vi "Process.vi"(8 "error in":errorcluster, 11 "Plugin in":refnum<class "Power Spectrum Density.lvclass">) -> (0 "error out":errorcluster, 3 "Plugin out":refnum<class "Power Spectrum Density.lvclass">)   [LabVIEW 2023, in "Power Spectrum Density.lvlib" / "Power Spectrum Density.lvclass"]
uses:
  Power Spectrum Density.lvclass
  Power Spectrum Density.lvclass/Power Spectrum Density.ctl
  Buffer Manager Function.ctl
  <vilib>/FlexLogger/SDK/PluginSDK.lvlibp/PEFClasses/SDK/Plugin/Plugin.lvclass
  C:/Program Files/National Instruments/LabVIEW 2023/vi.lib/FlexLogger/SDK/PluginSDK.lvlibp/PEFClasses/SDK/Plugin/Plugin.lvclass
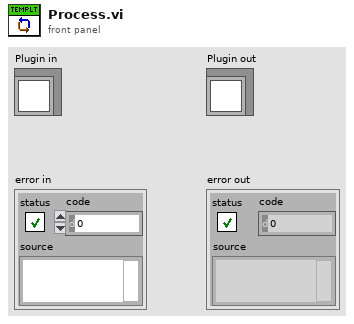
[diagram p1: front panel]
types:
  T1 = typedef "Power Spectrum Density.lvlib/Power Spectrum Density.lvclass/Buffer Manager Function.ctl" = enum16{"Get Data", "Buffer Data", "Reset Data"}
  T2 = typedef "Power Spectrum Density.lvlib/Power Spectrum Density.lvclass/Power Spectrum Density Data.ctl" = cluster{"First Time":bool, "Show PSD Window":bool, "Show PSD Window Clicked":bool, "Export mode":T3, "Window":T4, "dB":bool, "Averaging parameters":cluster{"averaging mode":enum16{"No averaging", "Vector averaging", "RMS averaging", "Peak hold"}, "weighting mode":enum16{"Linear", "Exponential"}, "number of averages":u32}, "Window parameter":dbl, "Number of Samples":i32, "PSD VI Ref":refnum<vi>}
  T3 = typedef "NI_MAPro.lvlib/Power Spectrum and PSD Export Mode.ctl" = u16
  T4 = typedef "NI_AALPro.lvlib/windowTd.ctl" = u32
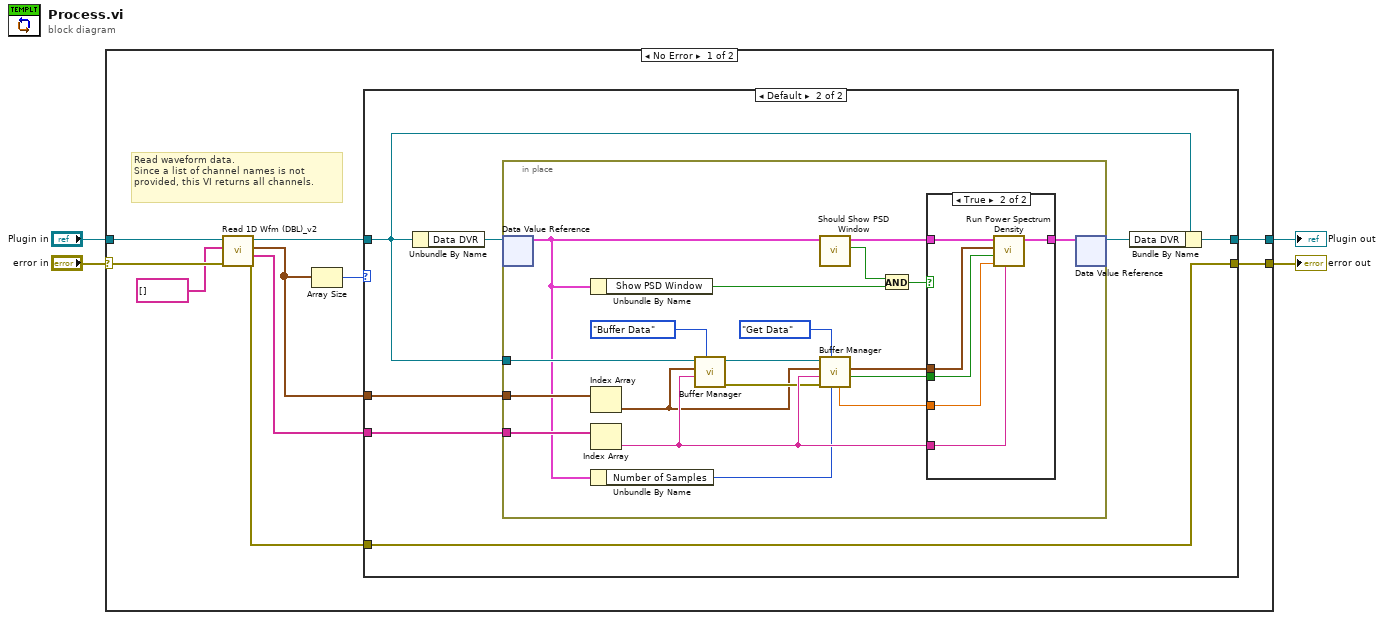
[diagram p0: block diagram]
diagram:
  n1 = case shown="No Error" "error in" {
    selector: "error in" -> [w13 w50]
    tunnel: [w11 w51] -> w3
    tunnel: "Plugin in" -> [w14 w51]
    tunnel: [w12 w50] -> w2
    frame No Error {
      # "Read waveform data.\nSince a list of channel names is not provided, this VI returns all channels."
      n2 = call <vilib>:"Read 1D Wfm (DBL)_v2.vi"("error in (no error)"=w13, "Unique Identifers (empty = all)"=string[] [] ("Unique Channel Identifers (empty = all)"), "Plugin in"=w14) -> ("error out"=w7:errorcluster, "Stream Names"=w5:string[], "Data"=w10:waveform(dbl)[], "Plugin out"=w8:refnum<class "Power Spectrum Density.lvclass">)  [unwired: 5 in]
      n3 = Array Size(array=w10) -> (size(s)=w9:i32)
      n4 = case shown="Default" w9 {
        tunnel: w10 -> [_ w23]
        tunnel: [w15 w22] -> w12
        tunnel: [w16 w18] -> w11
        tunnel: w8 -> [w16 w17]
        tunnel: w7 -> [w15 w22]
        tunnel: w5 -> [_ w21]
        frame 0 {
          # "No channels sending data to the plugin"
        }
        frame Default {
          n5 = Unbundle By Name(w17) -> ("Data DVR"=w20:refnum<data-value>)
          n6 = in-place {
            in-place-border: w23 -> [w40]
            in-place-border: w21 -> [w37]
            in-place-border: w17 -> [w39]
            n7 = in-place-dvr #1(w20) -> (w32:T2)  [unwired: 1 out]
            n8 = Unbundle By Name(w32) -> ("Show PSD Window"=w27:bool)
            n9 = Index Array(array=w40) -> (element=w29:waveform(dbl))  [unwired: 1 in]
            n10 = Index Array(array=w37) -> (element=w35:string)  [unwired: 1 in]
            n11 = Unbundle By Name(w32) -> ("Number of Samples"=w33:i32)
            n12 = call-dynamic "Buffer Manager.vi"("Function"=Buffer_Manager_Function."Buffer Data", "Unique Channel Identifier"=w35, "Waveform in"=w29, "Plugin in"=w39) -> ("error out"=w34:errorcluster, "Plugin out"=w36:refnum<class "Power Spectrum Density.lvclass">)  [unwired: 3 in, 3 out]
            n13 = call "Should Show PSD Window.vi"("Data in"=w32) -> ("Show window"=w26:bool, "Data out"=w42:T2)  [unwired: 9 in]
            n14 = call-dynamic "Buffer Manager.vi"("Number of Samples"=w33, "Function"=Buffer_Manager_Function."Get Data", "error in"=w34, "Unique Channel Identifier"=w35, "Waveform in"=w29, "Plugin in"=w36) -> ("Data Valid"=w25:bool, "Waveform out"=w28:waveform(dbl), "Percentage"=w24:dbl)  [unwired: 1 in, 2 out]
            n15 = And(x=w26, y=w27) -> (x .and. y?=w30:bool)
            n16 = case shown="True" w30 {
              tunnel: w42 -> [w43 w49]
              tunnel: [w43 w48] -> w41
              tunnel: w28 -> [_ w47]
              tunnel: w35 -> [_ w46]
              tunnel: w25 -> [_ w45]
              tunnel: w24 -> [_ w44]
              frame False {
              }
              frame True {
                n17 = call "Run Power Spectrum Density.vi"("Channel Name"=w46, "Percentage"=w44, "Data Valid"=w45, "Signal"=w47, "Data"=w49) -> ("Data out"=w48:T2)  [unwired: 6 in]
              }
            }
            n18 = in-place-dvr #1(w41) -> (w19:refnum<data-value>)  [unwired: 1 out]
          }
          n19 = Bundle By Name(cluster=w17, "Data DVR"=w19) -> (w18:refnum<class "Power Spectrum Density.lvclass">)
        }
      }
    }
    frame Error {
    }
  }
  "error out" <- w2
  "Plugin out" <- w3
